vi "Set User Info.vi"(9 "Password":string, 10 "Username":string, 11 "URI in":refnum<class "URI.lvclass">) -> (3 "URI out":refnum<class "URI.lvclass">)   [LabVIEW 2020, in "URI.lvlib" / "URI.lvclass"]
uses:
  URI.lvclass
  URI.lvclass/URI.ctl
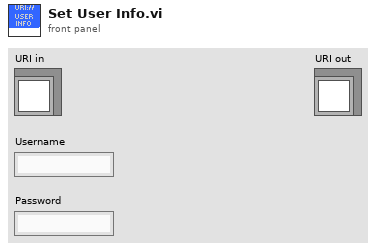
[diagram p1: front panel]
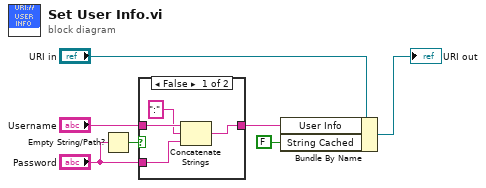
[diagram p0: block diagram]
diagram:
  n1 = Empty String/Path?(string/path="Password") -> (empty?=w6:bool)
  n2 = case shown="False" w6 {
    tunnel: "Password" -> [w10 _]
    tunnel: "Username" -> [w11 w12]
    tunnel: [w8 w12] -> w2
    frame False {
      n3 = Concatenate Strings(w11, ":" ("string"), w10) -> (w8:string)
    }
    frame True {
    }
  }
  n4 = Bundle By Name(cluster="URI in", "User Info"=w2, "String Cached"=FALSE) -> (→"URI out":refnum<class "URI.lvclass">)
